vi "ReadCANFrame.vi"(6 "Log Data?":bool, 8 "error in (no error)":errorcluster, 9 "timeout (0)":dbl format="%.2g", 10 "number to read (-1)":i32=-1, 11 "NI-XNET in":refnum<class "NI-XNET.lvclass">) -> (0 "error out":errorcluster, 2 "data":T1[](array[typedef]) {"payload" format="%x"; "timestamp" format="%<%.7X\n%x>T"; "type" items=["CAN Data"=0, "CAN Remote"=1, "CAN Bus Error"=2, "CAN 2.0 Data"=8, "CAN FD Data"=16, "CAN FD+BRS Data"=24, "J1939 Data"=192, "Delay"=224, "Log Trigger"=225, "Start Trigger"=226]; "identifier" format="%x"}, 3 "NI-XNET out":refnum<class "NI-XNET.lvclass">)   [LabVIEW 2023, in "HardwareAbstractionLayer_LVOOP.lvlib" / "CAN HAL Lib.lvlib" / "NI-XNET.lvclass"]
uses:
  NI-XNET.lvclass
  <vilib>/xnet/xnet.llb/XNET Frame CAN.ctl
  <vilib>/xnet/xnet.llb/XNET Frame Type CAN.ctl
  NI-XNET.lvclass/NI-XNET.ctl
  <vilib>/xnet/xnet.llb/XNET Read (Frame CAN).vi
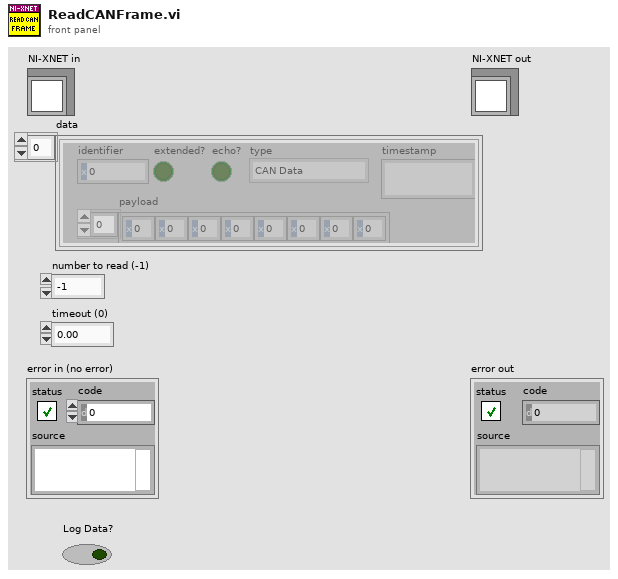
[diagram p1: front panel]
types:
  T1 = typedef "XNET Frame CAN.ctl" = cluster{"timestamp":timestamp, "payload":u8[], "identifier":u32, "type":T2, "extended?":bool, "echo?":bool}
  T2 = typedef "XNET Frame Type CAN.ctl" = u8
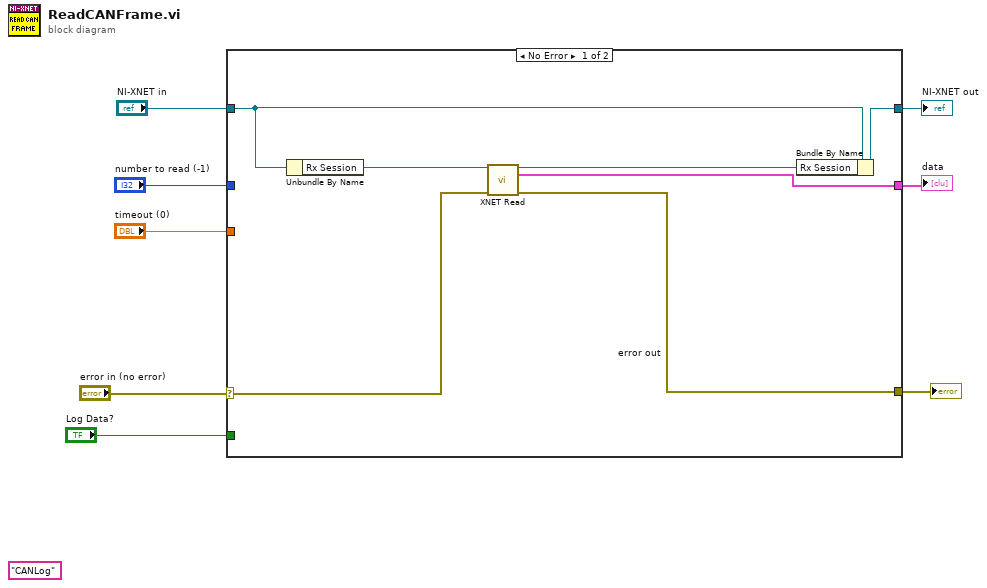
[diagram p0: block diagram]
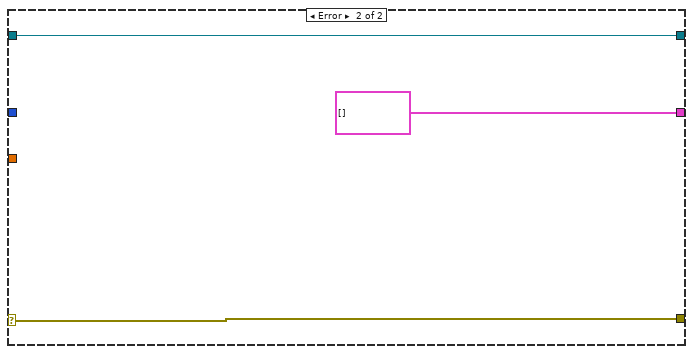
[diagram p2: hidden frame]
diagram:
  (unwired) "CANLog" ("name (unnamed)")
  n1 = case shown="No Error" "error in (no error)" {
    selector: "error in (no error)" -> [w11 w18]
    tunnel: [w9 w18] -> w3
    tunnel: [w13 w17] -> w5
    tunnel: "NI-XNET in" -> [w15 w17]
    tunnel: "timeout (0)" -> [_ _]
    tunnel: "number to read (-1)" -> [_ _]
    tunnel: [w10 T1[] [] ("data")] -> w4
    tunnel: "Log Data?" -> [_ _]
    frame No Error {
      n2 = Unbundle By Name(w15) -> ("Rx Session"=w14:refnum<k21>)
      n3 = call-poly <vilib>:"XNET Read.vi"("session in"=w14, "error in (no error)"=w11) -> ("session out"=w12:refnum<k21>, "data"=w10:T1[], "error out"=w9:errorcluster)  [unwired: 10 in, 1 out]
      n4 = Bundle By Name(cluster=w15, "Rx Session"=w12) -> (w13:refnum<class "NI-XNET.lvclass">)
    }
    frame Error {
    }
  }
  "error out" <- w3
  "NI-XNET out" <- w5
  "data" <- w4
